vi "verify WRITE SETUP parameters.vi"(8 "error in (no error)":errorcluster, 11 "Channel in":refnum<class "Channel.lvclass">) -> (0 "error out":errorcluster, 3 "Channel out":refnum<class "Channel.lvclass">)   [LabVIEW 2018, in "Channel.lvclass"]
uses:
  Channel.lvclass
  Channel.lvclass/Channel.ctl
  Simulated_CCD_Camera/Simulated Camera.lvclass/Simulated Camera.ctl
  Sim_Ixon_Ultra/Sim_Ixon_Ultra.lvclass
  C:/Users/Denis/Desktop/S4ACS/S4ACS/Simulated_CCD_Camera/Simulated Camera.lvclass
  Simulated_CCD_Camera/Simulated Camera.lvclass
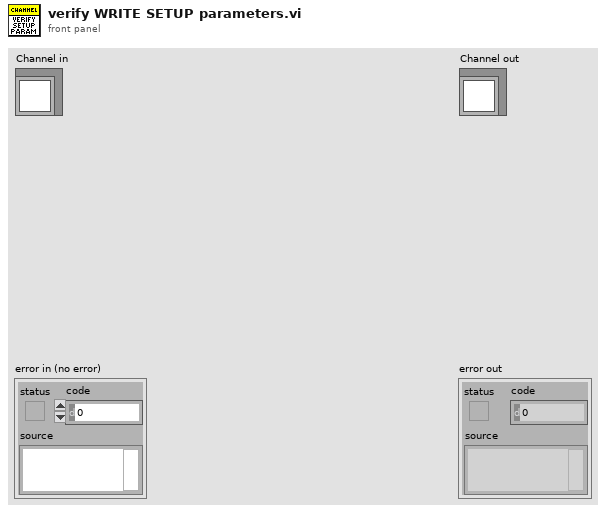
[diagram p1: front panel]
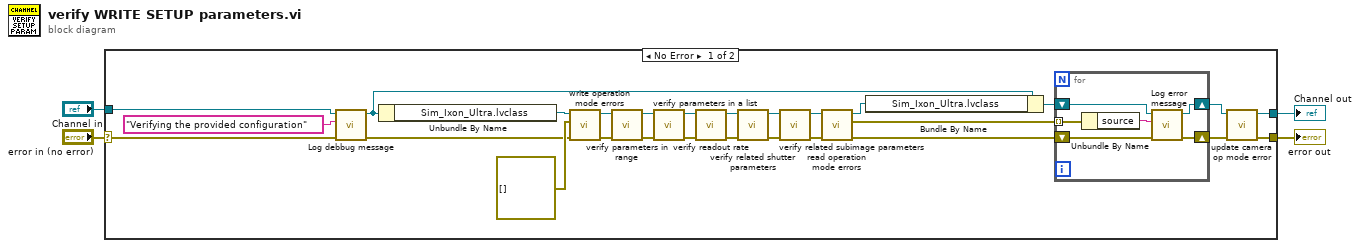
[diagram p0: block diagram]
diagram:
  n1 = case shown="No Error" "error in (no error)" {
    selector: "error in (no error)" -> [w17 w39]
    tunnel: [w26 w39] -> w3
    tunnel: [w27 w38] -> w1
    tunnel: "Channel in" -> [w20 w38]
    frame No Error {
      n2 = call "Log debbug message.vi"("error in (no error)"=w17, "String"="Verifying the provided configuration", "Channel in"=w20) -> ("error out"=w18:errorcluster, "Channel out"=w19:refnum<class "Channel.lvclass">)  [unwired: 7 in]
      n3 = Unbundle By Name(w19) -> ("Sim_Ixon_Ultra.lvclass"=w29:refnum<class "Sim_Ixon_Ultra.lvclass">)
      n4 = call "write operation mode errors.vi"("error in (no error)"=w18, "WRITE SETUP errors"=errorcluster[] [] ("Errors array"), "Simulated_CCD_Camera in"=w29) -> ("error out"=w30:errorcluster, "Simulated_CCD_Camera out"=w31:refnum<class "Sim_Ixon_Ultra.lvclass">)  [unwired: 7 in]
      n5 = call-dynamic "verify parameters in range.vi"("error in (no error)"=w30, "Simulated_CCD_Camera in"=w31) -> ("error out"=w11:errorcluster, "Simulated_CCD_Camera out"=w10:refnum<class "Sim_Ixon_Ultra.lvclass">)  [unwired: 8 in]
      n6 = call-dynamic "verify parameters in a list.vi"("error in (no error)"=w11, "Simulated_CCD_Camera in"=w10) -> ("error out"=w8:errorcluster, "Simulated_CCD_Camera out"=w5:refnum<class "Sim_Ixon_Ultra.lvclass">)  [unwired: 8 in]
      n7 = call "verify readout rate.vi"("error in (no error)"=w8, "Sim_Ixon_Ultra in"=w5) -> ("error out"=w7:errorcluster, "Sim_Ixon_Ultra out"=w6:refnum<class "Sim_Ixon_Ultra.lvclass">)  [unwired: 8 in]
      n8 = call "verify related shutter parameters.vi"("error in (no error)"=w7, "Simulated_CCD_Camera in"=w6) -> ("error out"=w12:errorcluster, "Simulated_CCD_Camera out"=w13:refnum<class "Sim_Ixon_Ultra.lvclass">)  [unwired: 8 in]
      n9 = call "verify related subimage parameters.vi"("error in (no error)"=w12, "Simulated_CCD_Camera in"=w13) -> ("error out"=w14:errorcluster, "Simulated_CCD_Camera out"=w15:refnum<class "Sim_Ixon_Ultra.lvclass">)  [unwired: 8 in]
      n10 = call "read operation mode errors.vi"("error in (no error)"=w14, "Simulated_CCD_Camera in"=w15) -> ("error out"=w25:errorcluster, "WRITE SETUP errors"=w24:errorcluster[], "Simulated_CCD_Camera out"=w9:refnum<class "Sim_Ixon_Ultra.lvclass">)  [unwired: 7 in]
      n11 = Bundle By Name(cluster=w19, "Sim_Ixon_Ultra.lvclass"=w9) -> (w22:refnum<class "Channel.lvclass">)
      n12 = for {
        shift-right: [w36] -> w21
        shift-left: w22 -> [w37]
        shift-right: [w35] -> w23
        shift-left: w25 -> [w34]
        tunnel: w24 -> [w33] mode=indexing
        n13 = Unbundle By Name(w33) -> ("source"=w32:string)
        n14 = call "Log error message.vi"("error in (no error)"=w34, "String"=w32, "Channel in"=w37) -> ("error out"=w35:errorcluster, "Channel out"=w36:refnum<class "Channel.lvclass">)  [unwired: 7 in]
      }
      n15 = call "update camera op mode error.vi"("error in (no error)"=w23, "Channel in"=w21) -> ("error out"=w26:errorcluster, "Channel out"=w27:refnum<class "Channel.lvclass">)  [unwired: 8 in]
    }
    frame Error {
    }
  }
  "error out" <- w3
  "Channel out" <- w1
